vi "Increment_Variables_MAIN.vi"(0 "Data Main":waveform(dbl)[](array[waveform]), 5 "Dummy Variable":dbl, 7 "On/Off":dbl, 9 "Operator Notes":string, 11 "error in 2":errorcluster, 12 "Speed Setpoint":dbl) -> (4 "Time Stamp":timestamp[](array[timestamp]), 6 "Dummy Variable Array":dbl[](array[numeric]), 10 "Operator Notes Array":string[](array[string]), 13 "On/Off Array":dbl[](array[numeric]), 14 "Speed Setpoint Array":dbl[](array[numeric]), 15 "error IO":errorcluster)   [LabVIEW 2016]
uses:
  <vilib>/Utility/error.llb/DialogType.ctl
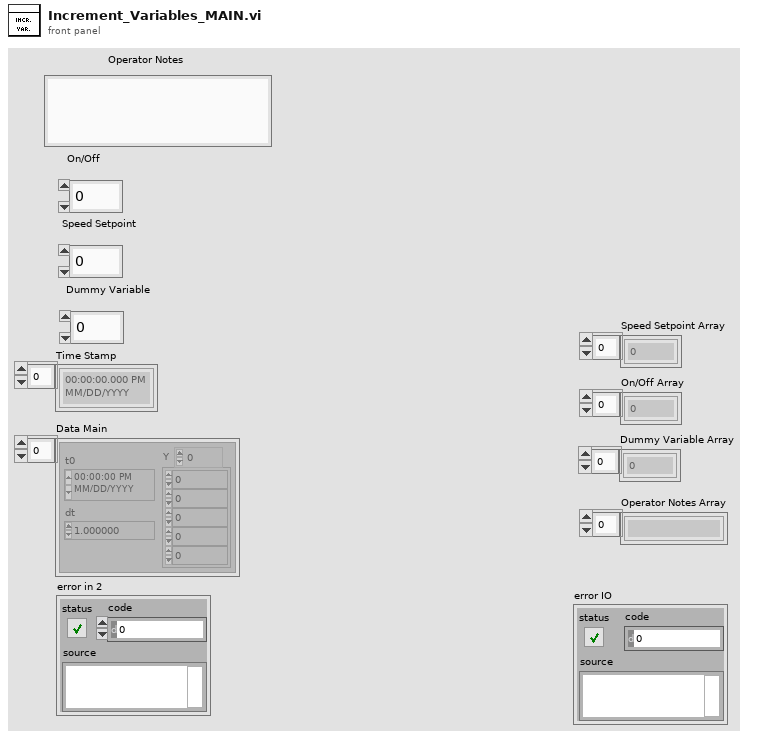
[diagram p1: front panel]
types:
  T1 = typedef "DialogType.ctl" = u16
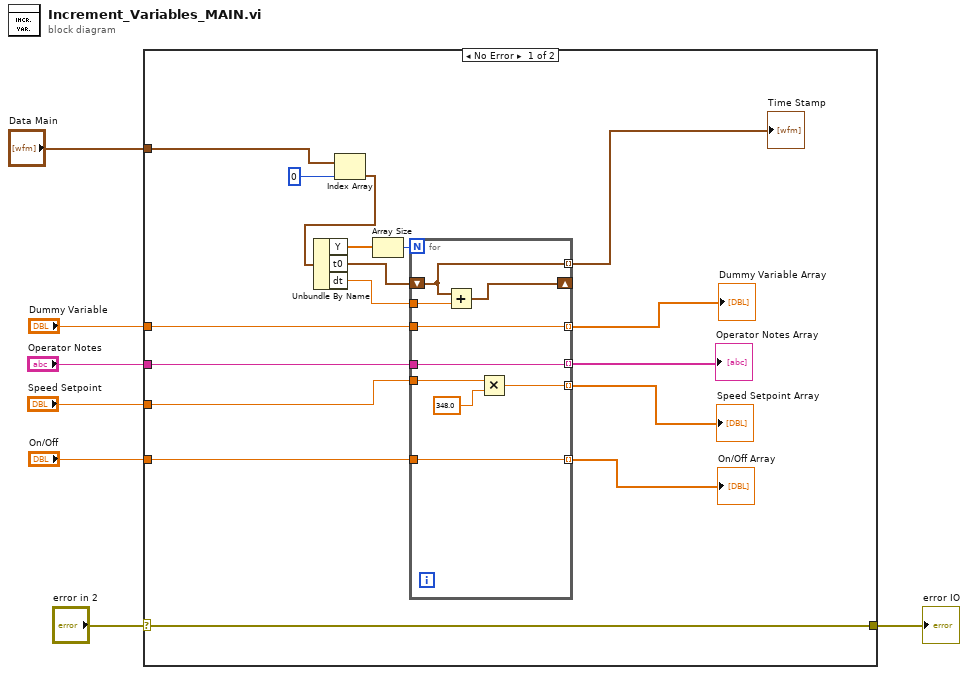
[diagram p0: block diagram]
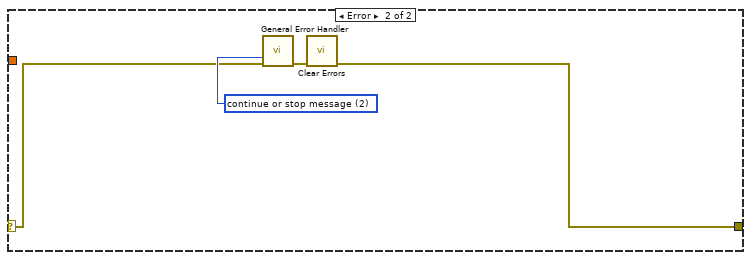
[diagram p2: hidden frame]
diagram:
  n1 = case shown="No Error" "error in 2" {
    selector: "error in 2" -> [w15 w35]
    tunnel: "Dummy Variable" -> [w24 _]
    tunnel: "Data Main" -> [w21 _]
    tunnel: "Operator Notes" -> [w16 _]
    tunnel: [w15 w34] -> w3
    tunnel: "Speed Setpoint" -> [w14 _]
    tunnel: "On/Off" -> [w8 _]
    frame No Error {
      n2 = Index Array(array=w21, index=0) -> (element=w22:waveform(dbl))
      n3 = Unbundle By Name(w22) -> ("Y"=w17:dbl[], "t0"=w19:timestamp, "dt"=w20:dbl)
      n4 = Array Size(array=w17) -> (size(s)=w18:i32)
      n5 = for {
        N: w18 -> [_]
        tunnel: w20 -> [w33]
        shift-right: [w32] -> _
        shift-left: w19 -> [w29]
        tunnel: [w31] -> w13 mode=indexing
        tunnel: w24 -> [w31]
        tunnel: [w30] -> w11 mode=indexing
        tunnel: w16 -> [w30]
        tunnel: w14 -> [w27]
        tunnel: [w26] -> w12 mode=indexing
        tunnel: [w29] -> w10 mode=indexing
        tunnel: [w28] -> w9 mode=indexing
        tunnel: w8 -> [w28]
        n6 = Add(x=w29, y=w33) -> (x+y=w32:timestamp)
        n7 = Multiply(x=w27, y=348.0) -> (x*y=w26:dbl)
      }
      "Dummy Variable Array" <- w13
      "Operator Notes Array" <- w11
      "Speed Setpoint Array" <- w12
      "Time Stamp" <- w10
      "On/Off Array" <- w9
    }
    frame Error {
      w36 = T1 2 items=["no dialog", "OK message", "continue or stop message", "OK message + warnings", "continue/stop + warnings"] ("type of dialog (OK msg:1)")
      n8 = call <vilib>:"General Error Handler.vi"("type of dialog (OK msg:1)"=w36, "error in (no error)"=w35) -> ("error out"=w37:errorcluster)  [unwired: 9 in, 4 out]
      n9 = call <vilib>:"Clear Errors.vi"("error in (no error)"=w37) -> ("error out"=w34:errorcluster)  [unwired: 5 in, 1 out]
    }
  }
  "error IO" <- w3
